vi "Parse Path Name.vi"(7 "PG Path":string) -> (4 "Table path":string, 6 "Column path":string, 8 "Table name":string, 10 "Column name":string, 15 "Column units":string)   [LabVIEW 2016, in "LV-Data.PGSQL.lvclass"]
uses:
  LV-Data.PGSQL.lvclass
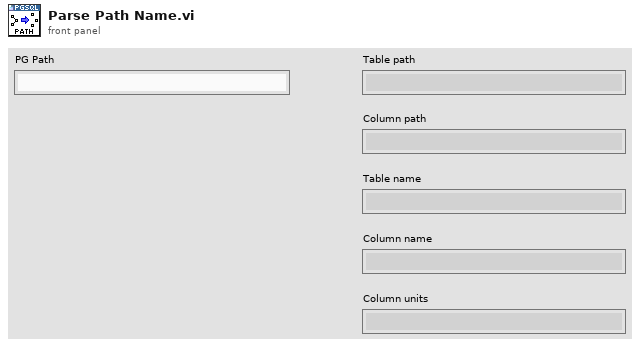
[diagram p1: front panel]
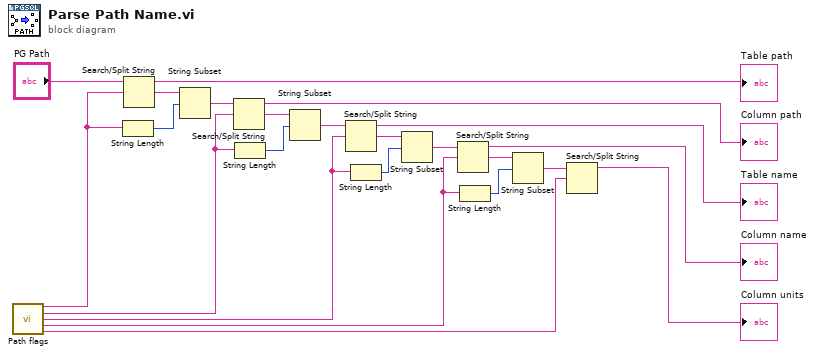
[diagram p0: block diagram]
diagram:
  n1 = call "Path flags.vi"() -> ("table_path()column_path"=w17:string, "column_path()table_name"=w14:string, "table_name()column_name"=w12:string, "column_name()units"=w8:string, "units()"=w2:string)  [unwired: 11 in]
  n2 = String Length(string=w17) -> (length=w16:i32)
  n3 = Search/Split String(string="PG Path", search string/char (-)=w17) -> (substring before match=→"Table path":string, match + rest of string=w21:string)  [unwired: 1 in, 1 out]
  n4 = String Subset(string=w21, offset (0)=w16) -> (substring=w20:string)  [unwired: 1 in]
  n5 = Search/Split String(string=w20, search string/char (-)=w14) -> (substring before match=→"Column path":string, match + rest of string=w15:string)  [unwired: 1 in, 1 out]
  n6 = String Length(string=w14) -> (length=w13:i32)
  n7 = String Subset(string=w15, offset (0)=w13) -> (substring=w18:string)  [unwired: 1 in]
  n8 = Search/Split String(string=w18, search string/char (-)=w12) -> (substring before match=→"Table name":string, match + rest of string=w11:string)  [unwired: 1 in, 1 out]
  n9 = String Length(string=w12) -> (length=w10:i32)
  n10 = String Subset(string=w11, offset (0)=w10) -> (substring=w9:string)  [unwired: 1 in]
  n11 = Search/Split String(string=w9, search string/char (-)=w8) -> (substring before match=→"Column name":string, match + rest of string=w7:string)  [unwired: 1 in, 1 out]
  n12 = String Length(string=w8) -> (length=w6:i32)
  n13 = String Subset(string=w7, offset (0)=w6) -> (substring=w3:string)  [unwired: 1 in]
  n14 = Search/Split String(string=w3, search string/char (-)=w2) -> (substring before match=→"Column units":string)  [unwired: 1 in, 2 out]
